vi "getUserInput.vi"(8 "error in (no error)":errorcluster, 10 "clickedLEDReference":refnum<vi>, 11 "Simon_Engine in":refnum<class "Simon_Engine.lvclass">) -> (0 "error out":errorcluster, 3 "Simon_Engine out":refnum<class "Simon_Engine.lvclass">)   [LabVIEW 2019, in "Simon_Engine.lvclass"]
doc: "This VI processes User's input by telling the Engine what was the clicked LED."
uses:
  Simon_Engine.lvclass
  Simon_Engine.lvclass/Simon_Engine.ctl
  LED/LED Class/LED.lvclass
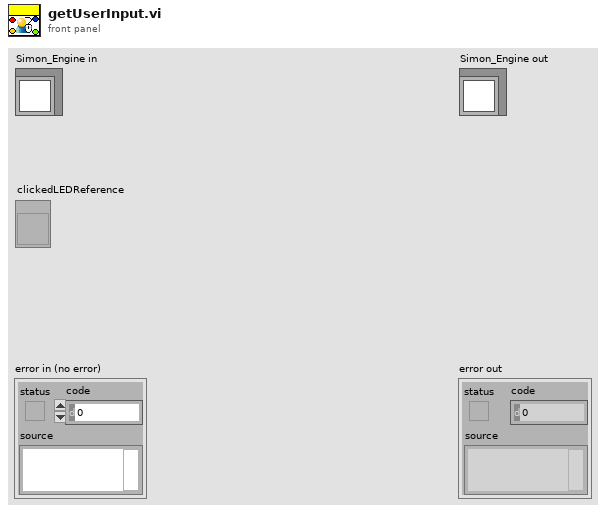
[diagram p1: front panel]
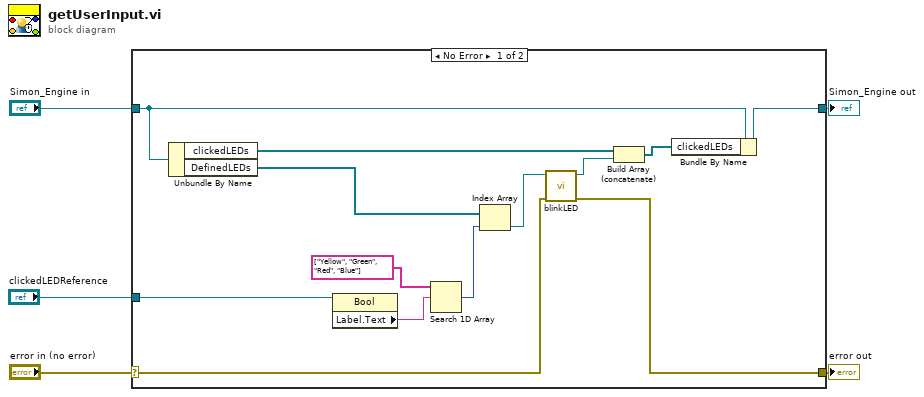
[diagram p0: block diagram]
diagram:
  n1 = case shown="No Error" "error in (no error)" {
    selector: "error in (no error)" -> [w10 w20]
    tunnel: [w11 w20] -> w4
    tunnel: [w9 w19] -> w2
    tunnel: "Simon_Engine in" -> [w14 w19]
    tunnel: "clickedLEDReference" -> [w12 _]
    frame No Error {
      n2 = Unbundle By Name(w14) -> ("clickedLEDs"=w7:refnum<class "LED.lvclass">[], "DefinedLEDs"=w13:refnum<class "LED.lvclass">[])
      n3 = property class="Bool"(reference=w12) -> ("Label.Text"=w16:string)  [unwired: 1 in, 2 out]
      n4 = Search 1D Array(1D array=string[] ["Yellow", "Green", "Red", "Blue"], element=w16) -> (index of element=w17:i32)  [unwired: 1 in]
      n5 = Index Array(array=w13, index=w17) -> (element=w18:refnum<class "LED.lvclass">)
      n6 = call "blinkLED.vi"("error in (no error)"=w10, "LED in"=w18) -> ("error out"=w11:errorcluster, "LED out"=w6:refnum<class "LED.lvclass">)  [unwired: 8 in]
      n7 = Build Array (concatenate)(w7, w6) -> (w8:refnum<class "LED.lvclass">[])
      n8 = Bundle By Name(cluster=w14, "clickedLEDs"=w8) -> (w9:refnum<class "Simon_Engine.lvclass">)
    }
    frame Error {
    }
  }
  "error out" <- w4
  "Simon_Engine out" <- w2
